vi "DequeueMessage.vi"(8 "error in (no error)":errorcluster, 11 "queue in":refnum<data-value>) -> (0 "error out":errorcluster, 1 "timeout":bool, 2 "message":variant, 3 "queue out":refnum<data-value>)   [LabVIEW 2009, in "PriorityQueue.lvlib"]
uses:
  PriorityQueue.lvlib
  PriorityQueue/PriorityQueue.lvclass
  LinkedList/position.ctl
  PriorityNode/PriorityNode.lvclass
  LLNode/LLNode.lvclass
  LinkedList/LinkedList.lvclass
  Message/Message.lvclass
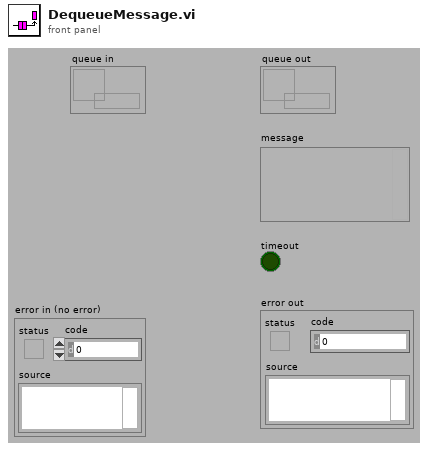
[diagram p1: front panel]
types:
  T1 = typedef "LinkedList.lvclass/position.ctl" = enum16{"Front", "Back", "Search"}
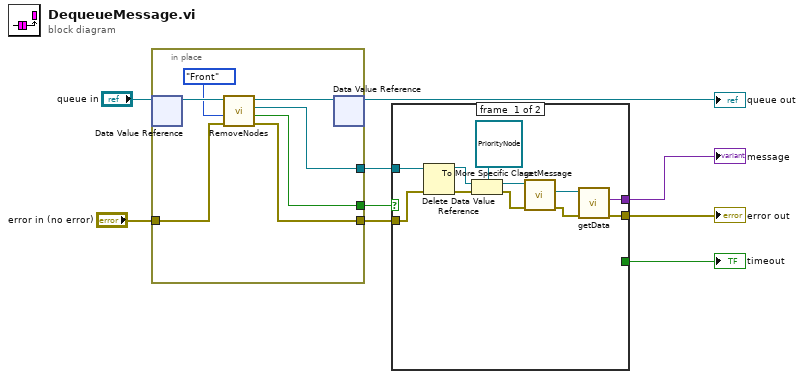
[diagram p0: block diagram]
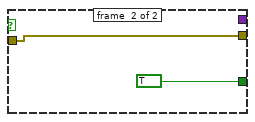
[diagram p2: hidden frame]
diagram:
  n1 = in-place {
    in-place-border: [w12] -> w4
    in-place-border: "error in (no error)" -> [w14]
    in-place-border: [w11] -> w7
    in-place-border: [w10] -> w6
    n2 = in-place-dvr #1("queue in") -> (w16:refnum<class "PriorityQueue.lvclass">)  [unwired: 1 out]
    n3 = call "RemoveNodes.vi"("error in (no error)"=w14, "position"=position."Front", "LinkedList in"=w16) -> ("error out"=w12:errorcluster, "ignored"=w11:bool, "RemovedNode"=w10:refnum<data-value>, "LinkedList out"=w13:refnum<class "PriorityQueue.lvclass">)  [unwired: 5 in]
    n4 = in-place-dvr #1(w13) -> (→"queue out":refnum<data-value>)  [unwired: 1 out]
  }
  n5 = case shown="True" w7 {
    tunnel: w6 -> [w26 _]
    tunnel: w4 -> [w27 w29]
    tunnel: [w18 w29] -> w3
    tunnel: [w17 _] -> w2
    tunnel: [_ TRUE] -> w1
    frame #0 {
      n6 = Delete Data Value Reference(data value reference=w26, error in=w27) -> (data value=w24:refnum<class "LLNode.lvclass">, error out=w25:errorcluster)
      n7 = To More Specific Class(target class=refnum<class "PriorityNode.lvclass"> refnum ("PriorityNode in"), reference=w24, error in=w25) -> (specific class reference=w22:refnum<class "PriorityNode.lvclass">, error out=w21:errorcluster)
      n8 = call "getMessage.vi"("error in (no error)"=w21, "PriorityNode in"=w22) -> ("error out"=w19:errorcluster, "Message.lvclass"=w20:refnum<class "Message.lvclass">)  [unwired: 7 in, 1 out]
      n9 = call "getData.vi"("error in (no error)"=w19, "Message in"=w20) -> ("error out"=w18:errorcluster, "Data"=w17:variant)  [unwired: 7 in, 1 out]
    }
    frame #1 {
    }
  }
  "error out" <- w3
  "timeout" <- w1
  "message" <- w2
